vi "Get Transform Matrix.vi"(8 "error in (no error)":errorcluster, 9 "Glyph Size":cluster{"Width":sgl, "Height":sgl}, 10 "Canvas Size":cluster{"Width":i32, "Height":i32}, 11 "Transform in":refnum<class "Transform.lvclass">) -> (0 "error out":errorcluster, 2 "Transform":T1, 3 "Transform out":refnum<class "Transform.lvclass">)   [LabVIEW 2023, in "Glyph Drawer.lvlib" / "Transform.lvclass"]
uses:
  Transform.lvclass
  <vilib>/Analysis/Matrix/Datatypes/RealMatrix.ctl
  <vilib>/Analysis/baseanly.llb/Real A x B.vi
  Glyph Drawer.lvlib
  <vilib>/Analysis/Matrix/NI_Matrix.lvlib
  <vilib>/Analysis/NI_AALBase.lvlib
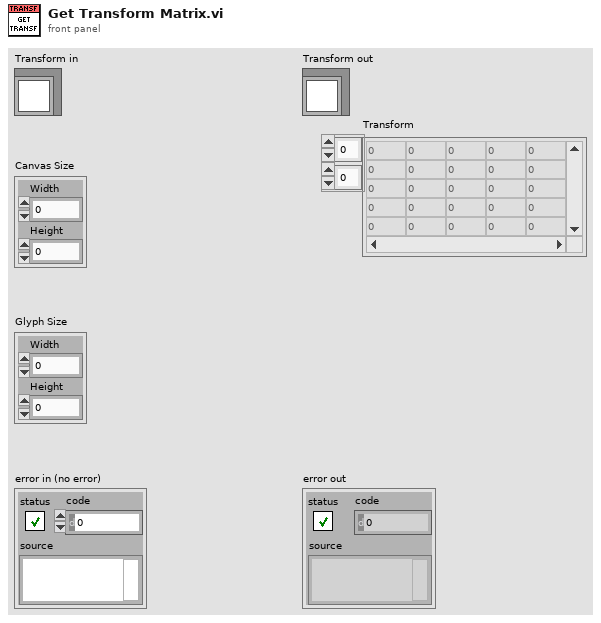
[diagram p1: front panel]
types:
  T1 = typedef "NI_Matrix.lvlib/RealMatrix.ctl" = dbl[][]
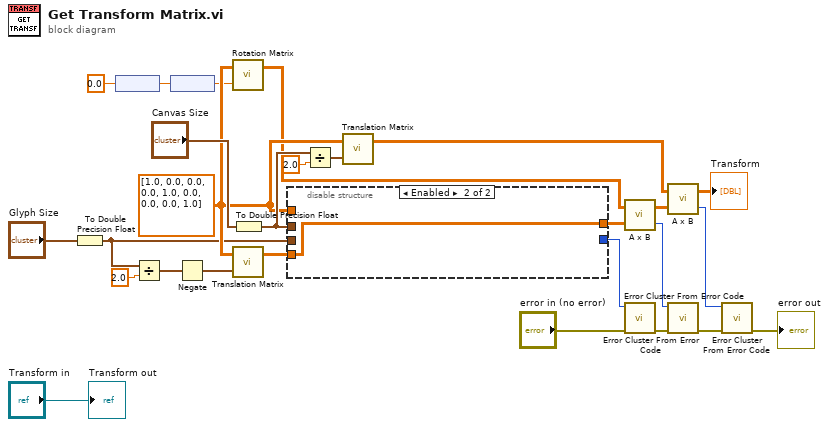
[diagram p0: block diagram]
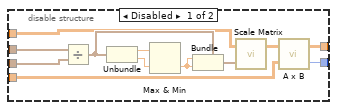
[diagram p2: hidden frame]
diagram:
  w21 = T1 [[1.0, 0.0, 0.0], [0.0, 1.0, 0.0], [0.0, 0.0, 1.0]] ("Matrix Type (2x2)")
  n1 = To Double Precision Float(number="Glyph Size") -> (double precision float=w1:cluster{"Width":dbl, "Height":dbl})
  n2 = node(0.0 ("Rotation")) -> (w10:dbl[unit])
  n3 = Divide(x=w1, y=2.0) -> (x/y=w18:cluster{"Width":dbl, "Height":dbl})
  n4 = node(w10) -> (w9:dbl)
  n5 = Negate(x=w18) -> (-x=w17:cluster{"Width":dbl, "Height":dbl})
  n6 = call "Rotation Matrix.vi"("Rotation rad"=w9, "Matrix Type (2x2)"=w21) -> ("Matrix Out"=w14:T1)  [unwired: 1 in]
  n7 = call "Translation Matrix.vi"("Translation"=w17, "Matrix Type (2x3)"=w21) -> ("Matrix Out"=w16:T1)  [unwired: 1 in]
  n8 = To Double Precision Float(number="Canvas Size") -> (double precision float=w23:cluster{"Width":dbl, "Height":dbl})
  n9 = disable-structure shown="Enabled" {
    disable-tunnel: w23 -> [w39 _]
    disable-tunnel: w21 -> [w33 _]
    disable-tunnel: w16 -> [w32 w40]
    disable-tunnel: [w30 w40] -> w15
    disable-tunnel: [w29 _] -> w7
    disable-tunnel: w1 -> [w28 _]
    frame Disabled {
      n10 = Divide(x=w39, y=w28) -> (x/y=w38:cluster{"Width":dbl, "Height":dbl})
      n11 = Unbundle(w38) -> ("Width"=w37:dbl, "Height"=w36:dbl)
      n12 = Max & Min(x=w37, y=w36) -> (min(x,y)=w35:dbl)  [unwired: 1 out]
      n13 = Bundle(cluster=w38, "Width"=w35, "Height"=w35) -> (w34:cluster{"Width":dbl, "Height":dbl})
      n14 = call "Scale Matrix.vi"("Scale"=w34, "Matrix Type (2x2)"=w33) -> ("Matrix Out"=w31:T1)  [unwired: 1 in]
      n15 = call-poly <vilib>:"A x B.vi"("B"=w32, "A"=w31) -> ("error"=w29:i32, "A x B"=w30:T1)
    }
    frame Enabled {
    }
  }
  n16 = Divide(x=w23, y=2.0) -> (x/y=w25:cluster{"Width":dbl, "Height":dbl})
  n17 = call "Translation Matrix.vi"("Translation"=w25, "Matrix Type (2x3)"=w21) -> ("Matrix Out"=w12:T1)  [unwired: 1 in]
  n18 = call-poly <vilib>:"A x B.vi"("B"=w15, "A"=w14) -> ("error"=w6:i32, "A x B"=w13:T1)
  n19 = call <vilib>:"Error Cluster From Error Code.vi"("error in (no error)"="error in (no error)", "error code (0)"=w7) -> ("error out"=w4:errorcluster)  [unwired: 7 in]
  n20 = call-poly <vilib>:"A x B.vi"("B"=w13, "A"=w12) -> ("error"=w5:i32, "A x B"=→"Transform":T1)
  n21 = call <vilib>:"Error Cluster From Error Code.vi"("error in (no error)"=w4, "error code (0)"=w6) -> ("error out"=w3:errorcluster)  [unwired: 7 in]
  n22 = call <vilib>:"Error Cluster From Error Code.vi"("error in (no error)"=w3, "error code (0)"=w5) -> ("error out"=→"error out":errorcluster)  [unwired: 7 in]
  "Transform out" <- "Transform in"
